vi "RBFSampler.vi"(8 "error in":errorcluster caption="entrée d'erreur", 11 "RBFSampler":T1={"gamma"=1.0, "n_components"=100, "random_state"=-1} {"random_state" min=-1}) -> (0 "error out":errorcluster caption="sortie d'erreur", 3 "RBFSampler.lvclass":refnum<class "RBFSampler.lvclass">)   [LabVIEW 2020]
doc: "Approximates feature map of an RBF kernel by Monte Carlo approximation of its Fourier transform.\n\nIt implements a variant of Random Kitchen Sinks.\n\nParameters : \n\n- gamma : float\nParameter of RBF kernel: exp(-gamma * x^2)\n\n- n_components : int\nNumber of Monte Carlo samples per original feature. Equals the dimensionality of the computed feature space.\n\n- random_state : int, RandomState instance or None, optional (default=None=-1)\nPseudo-random number generator to control the generation of the random weights and random offset when fitting the training data. Pass an int for reproducible output across multiple function calls. \n\n\nMethods :\n\n- Fit : Fit the model with X. Samples random projection according to n_features.\n\nParameters : X : {array-like, sparse matrix}, shape (n_samples, n_features)\n Training data, where n_samples in the number of samples and n_features is the number of features.\n\n\n- Fit Transform : Fit to data, then transform it. Fits transformer to X and y with optional parameters fit_params and returns a transformed version of X.\n\nParameters : X : {array-like, sparse matrix, dataframe} of shape (n_samples, n_features)\n y : ndarray of shape (n_samples,), default=None\n Target values.\n\nReturns : X_new : ndarray array of shape (n_samples, n_features_new)\n Transformed array.\n\n\n- Transform : Apply the approximate feature map to X.\n\nParameters : X : {array-like, sparse matrix}, shape (n_samples, n_features)\n New data, where n_samples in the number of samples and n_features is the number of features.\n\nReturns : X_new : array-like, shape (n_samples, n_components)"
uses:
  RBFSampler.lvclass
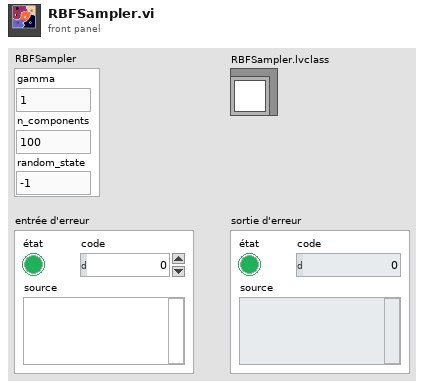
[diagram p1: front panel]
types:
  T1 = cluster{"gamma":dbl, "n_components":i32, "random_state":i32}
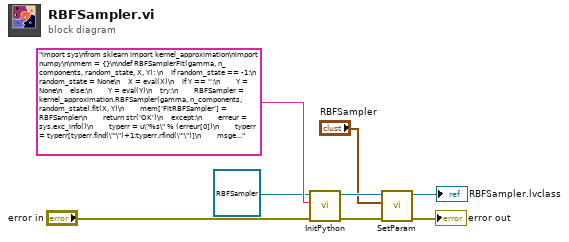
[diagram p0: block diagram]
diagram:
  n1 = call-dynamic "InitPython.vi"("error in (no error)"="error in", "Python Instruction"="import sys\nfrom sklearn import kernel_approximation\nimport numpy\n\nmem = {}\n\ndef RBFSamplerFit(gamma, n_components, random_state, X, Y): \n    if random_state == -1:\n        random_state = None\n    X = eval(X)\n    if Y == '':\n        Y = None\n    else:\n        Y = eval(Y)\n    try:\n        RBFSampler = kernel_approximation.RBFSampler(gamma, n_components, random_state).fit(X, Y)\n        mem['FitRBFSampler'] = RBFSampler\n        return str('OK')\n    except:\n        erreur = sys.exc_info()\n        typerr = u\"%s\" % (erreur[0])\n        typerr = typerr[typerr.find(\"'\")+1:typerr.rfind(\"'\")]\n        msgerr = u\"%s\" % (erreur[1])\n        message = str('/!\\\\ {0} : {1}'. format(typerr,msgerr))\n        return message \n\ndef RBFSamplerFitTransform(gamma, n_components, random_state, X, Y):\n    if random_state == -1:\n        random_state = None\n    X = eval(X)\n    if Y == '':\n        Y = None\n    else:\n        Y = eval(Y)\n    try:\n        RBFSampler = kernel_approximation.RBFSampler(gamma, n_components, random_state).fit_transform(X, Y)\n        RBFSampler = RBFSampler.tolist()\n        return str(RBFSampler)\n    except:\n        erreur = sys.exc_info()\n        typerr = u\"%s\" % (erreur[0])\n        typerr = typerr[typerr.find(\"'\")+1:typerr.rfind(\"'\")]\n        msgerr = u\"%s\" % (erreur[1])\n        message = str('/!\\\\ {0} : {1}'. format(typerr,msgerr))\n        return message \n    \n\ndef RBFSamplerTransform(gamma, n_components, random_state, X, Y):\n    if random_state == -1:\n        random_state = None\n    X = eval(X)\n    if Y == '':\n        Y = None\n    else:\n        Y = eval(Y)\n    try:\n        RBFSampler = mem['FitRBFSampler'].transform(X, Y)\n        RBFSampler = RBFSampler.tolist()\n        return str(RBFSampler)\n    except:\n        erreur = sys.exc_info()\n        typerr = u\"%s\" % (erreur[0])\n        typerr = typerr[typerr.find(\"'\")+1:typerr.rfind(\"'\")]\n        msgerr = u\"%s\" % (erreur[1])\n        message = str('/!\\\\ {0} : {1}'. format(typerr,msgerr))\n        return message", "Scikit-learn en entrée"=refnum<class "RBFSampler.lvclass"> refnum ("RBFSampler.lvclass")) -> ("error out"=w3:errorcluster, "Scikit-learn en sortie"=w5:refnum<class "RBFSampler.lvclass">)  [unwired: 7 in]
  n2 = call-dynamic "SetParam.vi"("error in (no error)"=w3, "RBFSampler"="RBFSampler", "RBFSampler.lvclass"=w5) -> ("error out"=→"error out":errorcluster, "RBFSampler.lvclass"=→"RBFSampler.lvclass":refnum<class "RBFSampler.lvclass">)  [unwired: 7 in]
